vi "SMU_Measurements.vi"(8 "Error In":errorcluster, 11 "Instrument_Visas":T2) -> (0 "Error Out":errorcluster, 1 "PI<0> Measurements":T1 {"current measurements" format="%#_6p"}, 2 "HV Measurements":T1 {"current measurements" format="%#_6p"}, 3 "Dut and Bridge Measurements":T1 {"current measurements" format="%#_6p"})   [LabVIEW 2013]
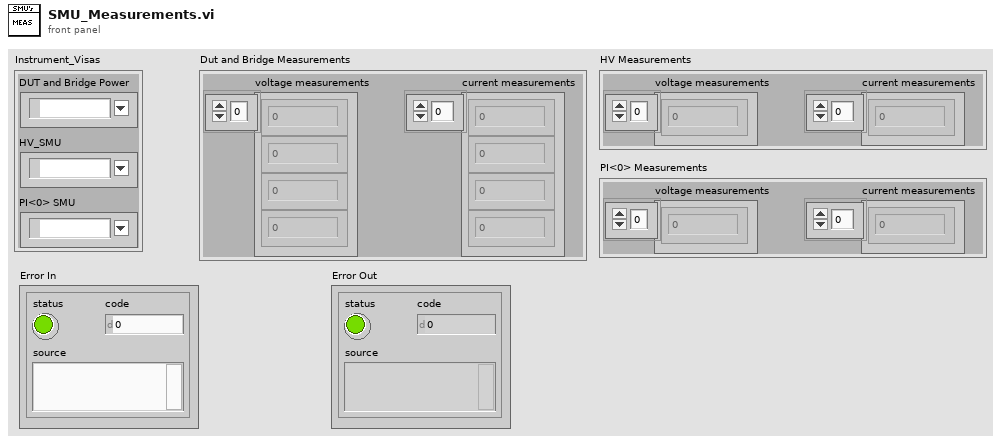
[diagram p1: front panel]
types:
  T1 = cluster{"voltage measurements":dbl[], "current measurements":dbl[]}
  T2 = cluster{"DUT and Bridge Power":refnum<k15>, "HV_SMU":refnum<k15>, "PI<0> SMU":refnum<k15>}
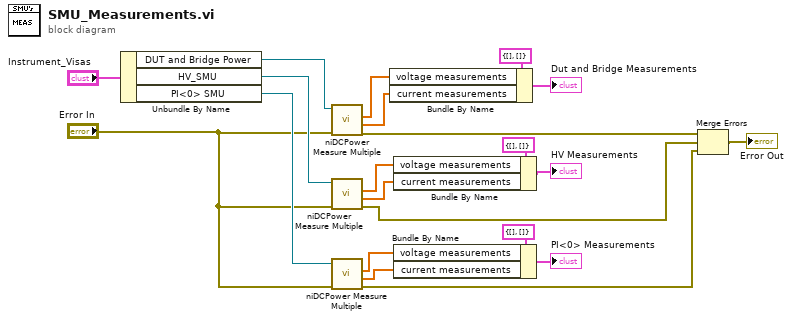
[diagram p0: block diagram]
diagram:
  n1 = Unbundle By Name("Instrument_Visas") -> ("DUT and Bridge Power"=w20:refnum<k15>, "HV_SMU"=w19:refnum<k15>, "PI<0> SMU"=w18:refnum<k15>)
  n2 = call <instrlib>:"niDCPower Measure Multiple.vi"("error in (no error)"="Error In", "instrument handle"=w20) -> ("error out"=w4:errorcluster, "current measurements"=w15:dbl[], "voltage measurements"=w16:dbl[])  [unwired: 6 in, 1 out]
  n3 = call <instrlib>:"niDCPower Measure Multiple.vi"("error in (no error)"="Error In", "instrument handle"=w19) -> ("error out"=w3:errorcluster, "current measurements"=w11:dbl[], "voltage measurements"=w12:dbl[])  [unwired: 6 in, 1 out]
  n4 = call <instrlib>:"niDCPower Measure Multiple.vi"("error in (no error)"="Error In", "instrument handle"=w18) -> ("error out"=w2:errorcluster, "current measurements"=w9:dbl[], "voltage measurements"=w10:dbl[])  [unwired: 6 in, 1 out]
  n5 = Bundle By Name(cluster=T1 {"voltage measurements"=[], "current measurements"=[]} ("Dut and Bridge Measurements"), "voltage measurements"=w16, "current measurements"=w15) -> (→"Dut and Bridge Measurements":T1)
  n6 = Bundle By Name(cluster=T1 {"voltage measurements"=[], "current measurements"=[]} ("Dut and Bridge Measurements"), "voltage measurements"=w12, "current measurements"=w11) -> (→"HV Measurements":T1)
  n7 = Bundle By Name(cluster=T1 {"voltage measurements"=[], "current measurements"=[]} ("Dut and Bridge Measurements"), "voltage measurements"=w10, "current measurements"=w9) -> (→"PI<0> Measurements":T1)
  n8 = Merge Errors(w4, w3, w2) -> (→"Error Out":errorcluster)
